vi "Format read string.vi"(8 "error in (no error)":errorcluster, 11 "Input String":string) -> (0 "error out":errorcluster, 3 "Formatted Output String":string)   [LabVIEW 2019, in "LabSSH.lvlib"]
doc: "<License>This software is distributed under the BSD 3-Clause License. For the full license please see license.txt or visit www.labvolution.com/license</License>"
uses:
  LabSSH.lvlib
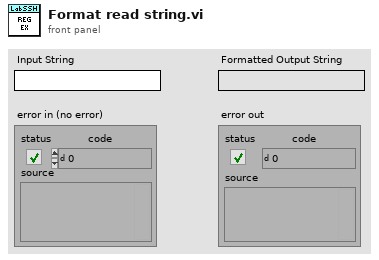
[diagram p1: front panel]
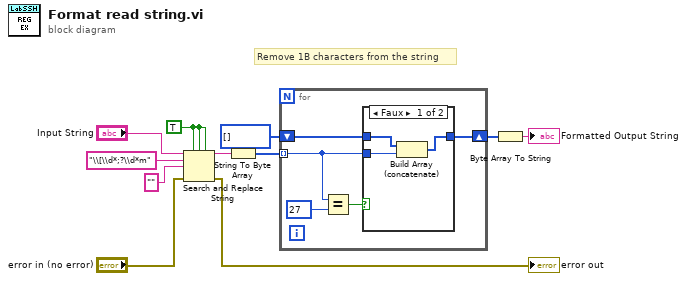
[diagram p0: block diagram]
diagram:
  w5 = TRUE ("replace all? (F)")
  # "Remove 1B characters from the string"
  n1 = Search and Replace String(replace all?=w5, case sensitive?=w5, multiline?=w5, input string="Input String", search string="\\[\\d*;?\\d*m" ("regular expression"), replace string="" ("replace string (\"\")"), error in="error in (no error)") -> (result string=w8:string, error out=→"error out":errorcluster)  [unwired: 1 in, 2 out]
  n2 = String To Byte Array(string=w8) -> (unsigned byte array=w9:u8[])
  n3 = for {
    tunnel: w9 -> [w14] mode=indexing
    shift-right: [w12] -> w10
    shift-left: u8[] [] -> [w13]
    n4 = Equal?(x=w14, y=u8 27) -> (x = y?=w15:bool)
    n5 = case shown="Faux" w15 {
      tunnel: w14 -> [w19 _]
      tunnel: w13 -> [w18 w20]
      tunnel: [w17 w20] -> w12
      frame False {
        n6 = Build Array (concatenate)(w18, w19) -> (w17:u8[])
      }
      frame True {
      }
    }
  }
  n7 = Byte Array To String(unsigned byte array=w10) -> (string=→"Formatted Output String":string)
